vi "S2DS_Filelog (SubVI).vi"(8 "error in":errorcluster, 10 "False channel":string[][](array[string]), 11 "path":path) -> (0 "error out":errorcluster)   [LabVIEW 2025]
uses:
  <vilib>/Utility/sysdir.llb/System Directory Type.ctl
  <vilib>/Utility/config.llb/Read Key (Path).vi
  <vilib>/Utility/config.llb/NI_LVConfig.lvlib
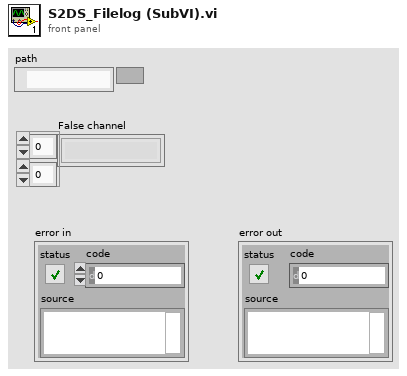
[diagram p1: front panel]
types:
  T1 = enum16{"open", "replace", "create", "open or create", "replace or create", "replace or create with confirmation"}
  T2 = typedef "System Directory Type.ctl" = i32
  T3 = typedef "NI_LVConfig.lvlib/Config Data RefNum.ctl" = refnum<k1>
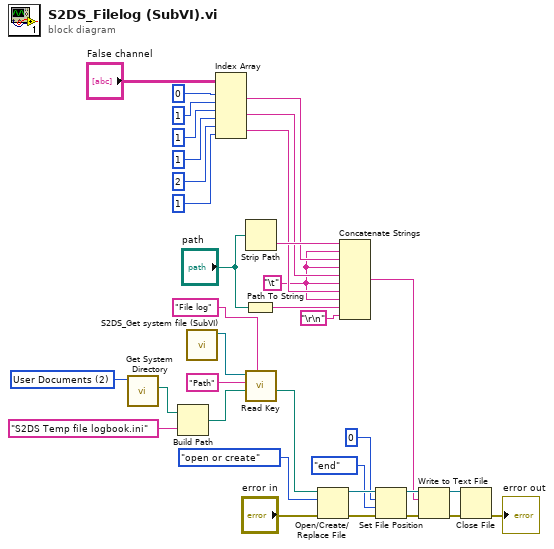
[diagram p0: block diagram]
diagram:
  w3 = "\t"
  w30 = T2 2 items=["User Home"=0, "User Desktop"=1, "User Documents"=2, "User Application Data"=3, "User Preferences"=4, "User Temporary"=5, "Public Documents"=6, "Public Application Data"=7, "Public Preferences"=8, "Public Cache"=13, "System Core Libraries"=9, "System Installed Libraries"=10, "Application Files"=11, "Boot Volume Root"=12] ("system directory type")
  n1 = call <vilib>:"Get System Directory.vi"("system directory type"=w30) -> ("system directory"=w31:path)  [unwired: 10 in]
  n2 = Build Path(base path=w31, name or relative path="S2DS Temp file logbook.ini") -> (appended path=w29:path)
  n3 = call "S2DS_Get system file (SubVI).vi"() -> ("Refnum out"=w35:T3)  [unwired: 10 in, 1 out]
  n4 = Index Array(array="False channel", index (row) #1=0 ("index (row)"), index (col) #1=1 ("disabled index (col)"), index (row) #2=1 ("index (row)"), index (col) #2=1 ("disabled index (col)"), index (row) #3=2 ("index (row)"), index (col) #3=1 ("disabled index (col)")) -> (element #1=w13:string, element #2=w5:string, element #3=w4:string)
  n5 = Path To String(path="path") -> (string=w2:string)
  n6 = Strip Path(path="path") -> (name=w16:string)  [unwired: 1 out]
  n7 = call-poly <vilib>:"Read Key.vi"("section"="File log", "default value"=w29, "key"="Path", "refnum"=w35) -> ("value"=w17:path)  [unwired: 4 in, 3 out]
  n8 = Open/Create/Replace File(file path (use dialog)=w17, error in="error in", operation (0:open)=T1."open or create") -> (refnum out=w25:refnum<file>, error out=w24:errorcluster)  [unwired: 3 in, 1 out]
  n9 = Concatenate Strings(w16, w3, w13, w3, w5, w3, w4, w3, w2, "\r\n") -> (w12:string)
  n10 = Set File Position(offset (in bytes) (0)=i64 0, refnum=w25, from (0:start)=enum16{"start", "end", "current"}."end", error in=w24) -> (refnum out=w22:refnum<file>, error out=w23:errorcluster)
  n11 = Write to Text File(file (use dialog)=w22, text=w12, error in=w23) -> (refnum out=w27:refnum<file>, error out=w28:errorcluster)  [unwired: 1 in, 1 out]
  n12 = Close File(refnum=w27, error in=w28) -> (error out=→"error out":errorcluster)  [unwired: 1 out]
